vi "floatToInt.vi"(1 "bits":u16, 2 "x_min":fxp<+/-,32,17>, 3 "x_max":fxp<+/-,32,17>, 4 "x":fxp<+/-,32,17>) -> (0 "Integer":u32 format="%x")   [LabVIEW 2019]
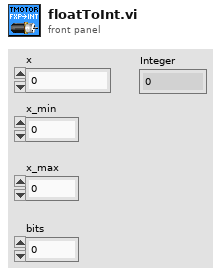
[diagram p1: front panel]
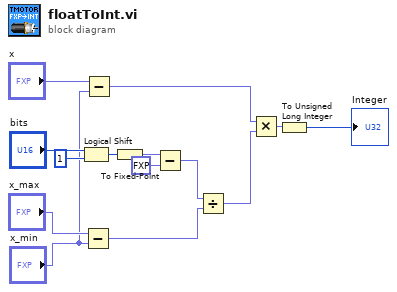
[diagram p0: block diagram]
diagram:
  n1 = Logical Shift(y="bits", x=u32 1) -> (x << y=w2:u32)
  n2 = Subtract(x="x_max", y="x_min") -> (x-y=w10:fxp<+,32,17>)
  n3 = Subtract(x="x", y="x_min") -> (x-y=w7:fxp<+/-,32,17>)
  n4 = To Fixed-Point(number=w2) -> (fixed-point=w1:fxp<+/-,32,17>)  [unwired: 1 in]
  n5 = Subtract(x=w1, y=fxp<+,1,2> 2.0) -> (x-y=w3:fxp<+/-,32,17>)
  n6 = Divide(x=w3, y=w10) -> (x/y=w6:fxp<+,32,17>)
  n7 = Multiply(x=w7, y=w6) -> (x*y=w5:fxp<+/-,32,17>)
  n8 = To Unsigned Long Integer(number=w5) -> (unsigned 32bit integer=→"Integer":u32)
